vi "Data Server Find Indexes from Variable Names.vi"(8 "Comand string":string, 11 "Variable names":string[](array[string])) -> (0 "Command error":bool, 3 "Index array":i32[](array[numeric]))   [LabVIEW 2011, in "Data Server VIs.lvlib"]
uses:
  Data Server VIs.lvlib
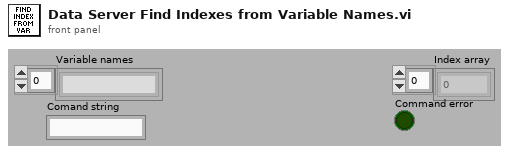
[diagram p1: front panel]
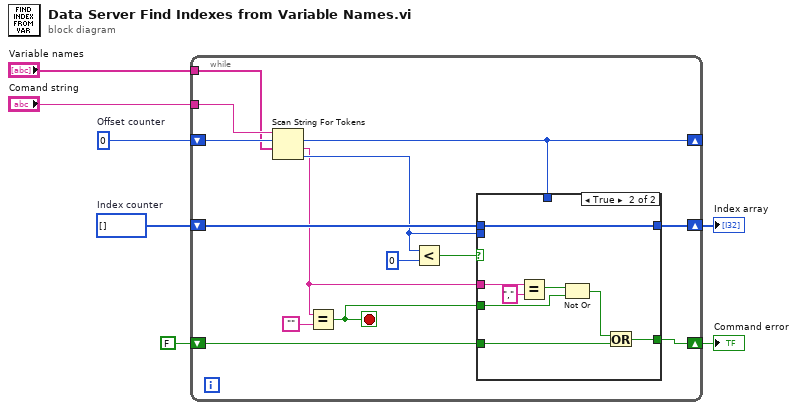
[diagram p0: block diagram]
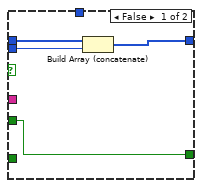
[diagram p2: hidden frame]
diagram:
  w6 = i32[] []  # Index counter
  w7 = 0  # Offset counter
  n1 = while {
    tunnel: "Comand string" -> [w16]
    shift-right: [w17] -> _
    shift-left: w7 -> [w21]
    shift-right: [w14] -> w2
    shift-left: w6 -> [w15]
    shift-right: [w10] -> w5
    shift-left: FALSE -> [w9]
    tunnel: "Variable names" -> [w8]
    stop <- w11 stop-if-true
    n2 = Scan String For Tokens(7:w8, 8:w21, 9:w16) -> (0:w13:i32, 1:w12:string, 2:w17:i32)  [unwired: 3 in, 1 out]
    n3 = Equal?(x=w12, y="") -> (x = y?=w11:bool)
    n4 = Less?(x=w13, y=0) -> (x < y?=w19:bool)
    n5 = case shown="True" w19 {
      tunnel: w13 -> [w24 _]
      tunnel: w17 -> [_ _]
      tunnel: w15 -> [w25 w33]
      tunnel: [w23 w33] -> w14
      tunnel: w12 -> [_ w32]
      tunnel: w11 -> [w22 w29]
      tunnel: [w22 w26] -> w10
      tunnel: w9 -> [_ w28]
      frame False {
        n6 = Build Array (concatenate)(w25, w24) -> (w23:i32[])
      }
      frame True {
        n7 = Equal?(x=w32, y=",") -> (x = y?=w30:bool)
        n8 = Not Or(1:w29, 2:w30) -> (0:w27:bool)
        n9 = Or(x=w27, y=w28) -> (x .or. y?=w26:bool)
      }
    }
  }
  "Index array" <- w2
  "Command error" <- w5
